vi "Switch Solenoid Feedthrough.vi"(8 "error in (no error)":errorcluster, 10 "Only Turn On (F)":bool, 11 "Main.lvlib:Main.lvclass":refnum<class "Main.lvclass">) -> (0 "error out":errorcluster, 3 "Actor out":refnum<class "Actor.lvclass">)   [LabVIEW 2018, in "Main.lvlib" / "Main.lvclass"]
uses:
  Main.lvclass
  C:/Program Files (x86)/National Instruments/LabVIEW 2018/vi.lib/ActorFramework/Actor/Actor.lvclass
  <vilib>/ActorFramework/Actor/Actor.lvclass
  Main.lvclass/Main.ctl
  Feeder Actor/Feeder Messages/Switch Solenoid Feedthrough Msg/Switch Solenoid Feedthrough Msg.lvclass/Switch Solenoid Feedthrough Msg.ctl
  <vilib>/ActorFramework/Message Enqueuer/Message Enqueuer.lvclass/Message Enqueuer.ctl
  <vilib>/ActorFramework/Message Enqueuer/Enqueue.vi
  Feeder Actor/Feeder Messages/Switch Solenoid Feedthrough Msg/Switch Solenoid Feedthrough Msg.lvclass
  C:/Program Files (x86)/National Instruments/LabVIEW 2018/vi.lib/ActorFramework/Message/Message.lvclass
  <vilib>/ActorFramework/Message Priority Queue/Priority Enqueue.vi
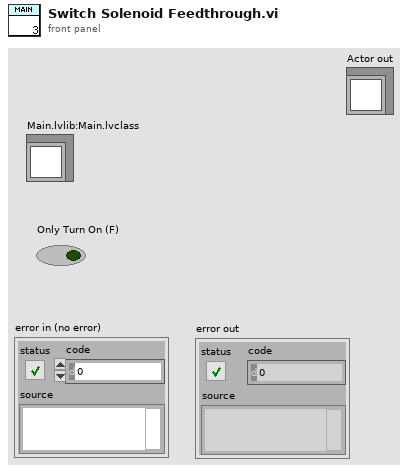
[diagram p1: front panel]
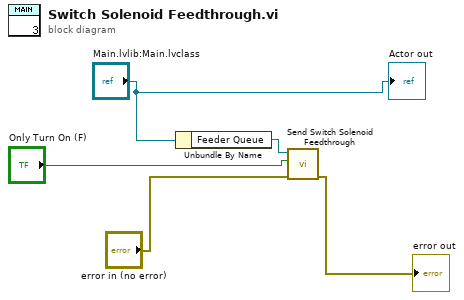
[diagram p0: block diagram]
diagram:
  n1 = Unbundle By Name("Main.lvlib:Main.lvclass") -> ("Feeder Queue"=w5:refnum<class "Message Enqueuer.lvclass">)
  n2 = call "Send Switch Solenoid Feedthrough.vi"("error in (no error)"="error in (no error)", "Only Turn On (F)"="Only Turn On (F)", "Message Enqueuer"=w5) -> ("error out"=→"error out":errorcluster)  [unwired: 7 in, 1 out]
  "Actor out" <- "Main.lvlib:Main.lvclass"
